vi "Visa Write data.vi"(8 "错误输入（无错误）":errorcluster, 10 "Write Data":string, 11 "VISA":T1={"VISA"="", "baud rate"=9600, "data bits"=8, "parity"=enum."None", "stop bits"=10, "flow control"=0} {"flow control" items=["无", "XON/XOFF", "RTS/CTS", "XON/XOFF & RTS/CTS", "DTR/DSR", "XON/XOFF & DTR/DSR"]; "stop bits" items=["1.0"=10, "1.5"=15, "2.0"=20]; "data bits" min=5 max=8 step=1}) -> (0 "error out":errorcluster caption="错误输出", 2 "State":bool, 3 "VISA Out":T1={"VISA"="", "baud rate"=9600, "data bits"=8, "parity"=enum."None", "stop bits"=10, "flow control"=0} {"flow control" items=["无", "XON/XOFF", "RTS/CTS", "XON/XOFF & RTS/CTS", "DTR/DSR", "XON/XOFF & DTR/DSR"]; "stop bits" items=["1.0"=10, "1.5"=15, "2.0"=20]; "data bits" min=5 max=8 step=1})   [LabVIEW 2014]
uses:
  <vilib>/Instr/_visa.llb/VISA Flush IO Buffer Mask.ctl
  Ctr/VISA Ctr.ctl
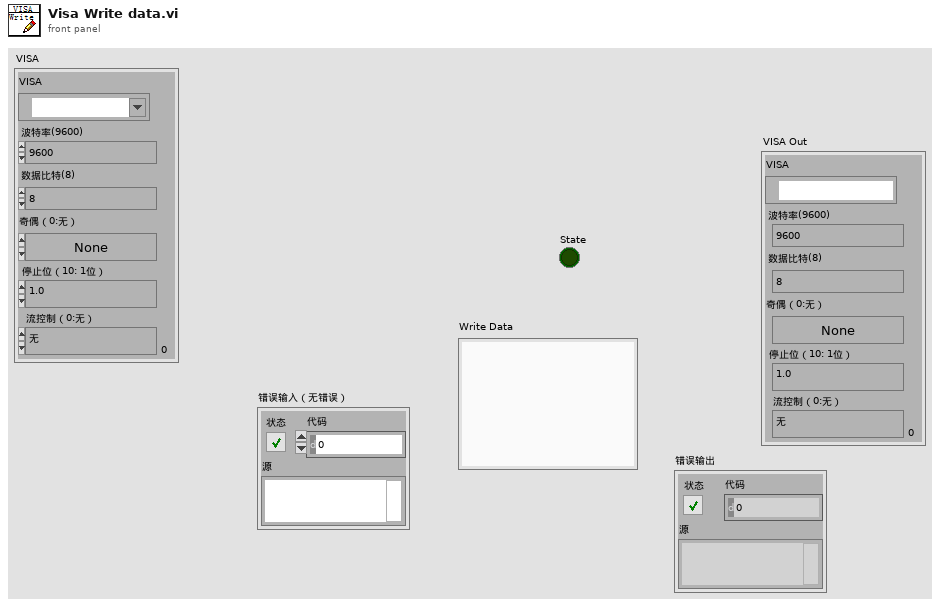
[diagram p1: front panel]
types:
  T1 = typedef "VISA Ctr.ctl" = cluster{"VISA":refnum<visa-resource-name>, "baud rate":u32, "data bits":u16, "parity":enum16{"None", "Odd", "Even", "Mark", "Space"}, "stop bits":u16, "flow control":u16}
  T2 = typedef "VISA Flush IO Buffer Mask.ctl" = u16
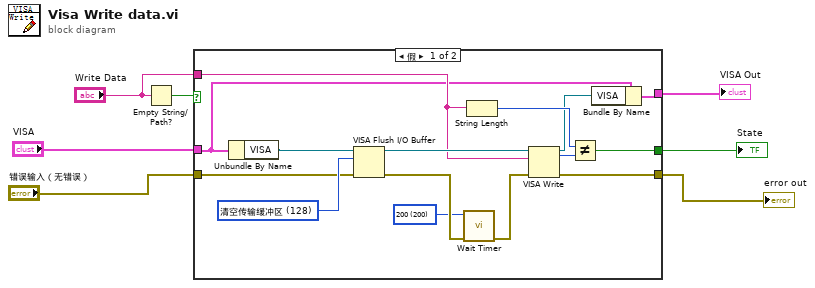
[diagram p0: block diagram]
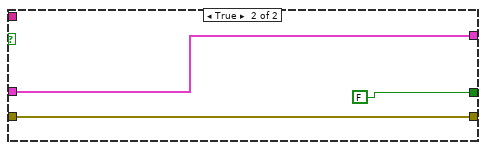
[diagram p2: hidden frame]
diagram:
  n1 = Empty String/Path?(string/path="Write Data") -> (empty?=w5:bool)
  n2 = case shown="假" w5 {
    tunnel: "VISA" -> [w10 w25]
    tunnel: "错误输入（无错误）" -> [w21 w24]
    tunnel: [w16 w24] -> w2
    tunnel: "Write Data" -> [w15 _]
    tunnel: [w8 w25] -> w1
    tunnel: [w12 FALSE] -> w3
    frame False {
      w19 = u16 200 items=["10"=10, "20"=20, "50"=50, "80"=80, "100"=100, "200"=200, "300"=300, "400"=400, "500"=500, "600"=600, "700"=700, "800"=800, "900"=900, "1000"=1000] ("Dely")
      w22 = T2 128 items=["清空接收缓冲区"=16, "向设备写入传输缓冲区"=32, "清空接收缓冲区（无I/O）"=64, "清空传输缓冲区"=128] ("Mask")
      n3 = Unbundle By Name(w10) -> ("VISA"=w11:refnum<visa-resource-name>)
      n4 = VISA Flush I/O Buffer(VISA resource name=w11, mask (16)=w22, error in (no error)=w21) -> (VISA resource name out=w17:refnum<visa-resource-name>, error out=w20:errorcluster)
      n5 = call "Wait Timer.vi"("error in (no error)"=w20, "Dely"=w19) -> ("error out"=w18:errorcluster)  [unwired: 8 in, 1 out]
      n6 = String Length(string=w15) -> (length=w13:i32)
      n7 = VISA Write(VISA resource name=w17, write buffer=w15, error in (no error)=w18) -> (VISA resource name out=w9:refnum<visa-resource-name>, return count=w14:u32, error out=w16:errorcluster)
      n8 = Not Equal?(x=w13, y=w14) -> (x != y?=w12:bool)
      n9 = Bundle By Name(cluster=w10, "VISA"=w9) -> (w8:T1)
    }
    frame True {
    }
  }
  "VISA Out" <- w1
  "State" <- w3
  "error out" <- w2
